vi "test frame felica psk.vi"() -> ()   [LabVIEW 2019]
uses:
  <vilib>/Analysis/3filter.llb/Filter Passband Type.ctl
  <vilib>/addons/Modulation/Analog/controls/Complex Data Waveform.ctl
  <vilib>/addons/Modulation/Analog/support/mod_Set Error Source.vi
  <vilib>/addons/Modulation/Digital/Support/Common/Validators/mod_Generate Filter Coefficients Validate.vi
  <vilib>/addons/Modulation/Digital/General/subVIs/mod_Generate Filter Coefficients.vi
  <vilib>/addons/Modulation/Digital/General/MT Generate PSK System Parameters(M).vi
  <vilib>/Waveform/DWDTOps.llb/DWDT Binary U8 to Digital.vi
  <vilib>/addons/Modulation/Analog/MT Upconvert Baseband (Real).vi
  <vilib>/addons/Modulation/Analog/MT Downconvert Passband (Real).vi
  <vilib>/express/express analysis/Spectral/Block/exnSpectralBlock spectral measurements RMS poly.vi
  <vilib>/express/express analysis/Spectral/Block/exnSpectralBlock spectral measurements RMS WFM.vi
  <vilib>/Analysis/3filter.llb/Butterworth Filter (DBL).vi
  <vilib>/express/express analysis/Spectral/XNode/ExpressSpectralMeasurementsBlockNode.xnode
  <vilib>/addons/Modulation/niDMT.lvlib
  <vilib>/addons/Modulation/niAMT.lvlib
  <vilib>/Analysis/NI_AALBase.lvlib
panel:
  out "Analog signal 4":waveform(dbl)(graph)
  out "spectrum analog signal 5":cluster{"t0":dbl, "dt":dbl, "Y":dbl[]}(graph)
  out "spectrum analog signal 4":cluster{"t0":dbl, "dt":dbl, "Y":dbl[]}(graph)
  out "ripple":dbl format="%.2p"
  out "output array":i16[](array[numeric])
  out "output bit stream":i8[](array[numeric])
  out "Analog signal 3":waveform(dbl)(graph)
  in  "command":enum16{"WUP_REQ"}(ring)
  out "error":i32
  out "spectrum analog signal 3":cluster{"t0":dbl, "dt":dbl, "Y":dbl[]}(graph)
  out "Analog signal 2":waveform(dbl)(graph)
  out "spectrum analog signal 2":cluster{"t0":dbl, "dt":dbl, "Y":dbl[]}(graph)
  out "spectrum analog signal":cluster{"t0":dbl, "dt":dbl, "Y":dbl[]}(graph)
  in  "CARRIER (hz)":dbl
  in  "BIT RATE":dbl
  out "LENGHT":u8[](array[numeric]) format="%x"
  out "dt":dbl
  out "Analog signal":waveform(dbl)(graph)
  out "video signal":cluster{"t0":dbl, "dt":dbl, "Y":dbl[]}(graph)
  out "Digital SIGNAL":digitalwaveform(graph)
  out "CRC":u8[](array[numeric]) format="%x"
  in  "Data":u8[](array[numeric]) format="%x"
  in  "SYNC":u8[](array[numeric]) format="%x"
  in  "Preambula":u8[](array[numeric]) format="%x"
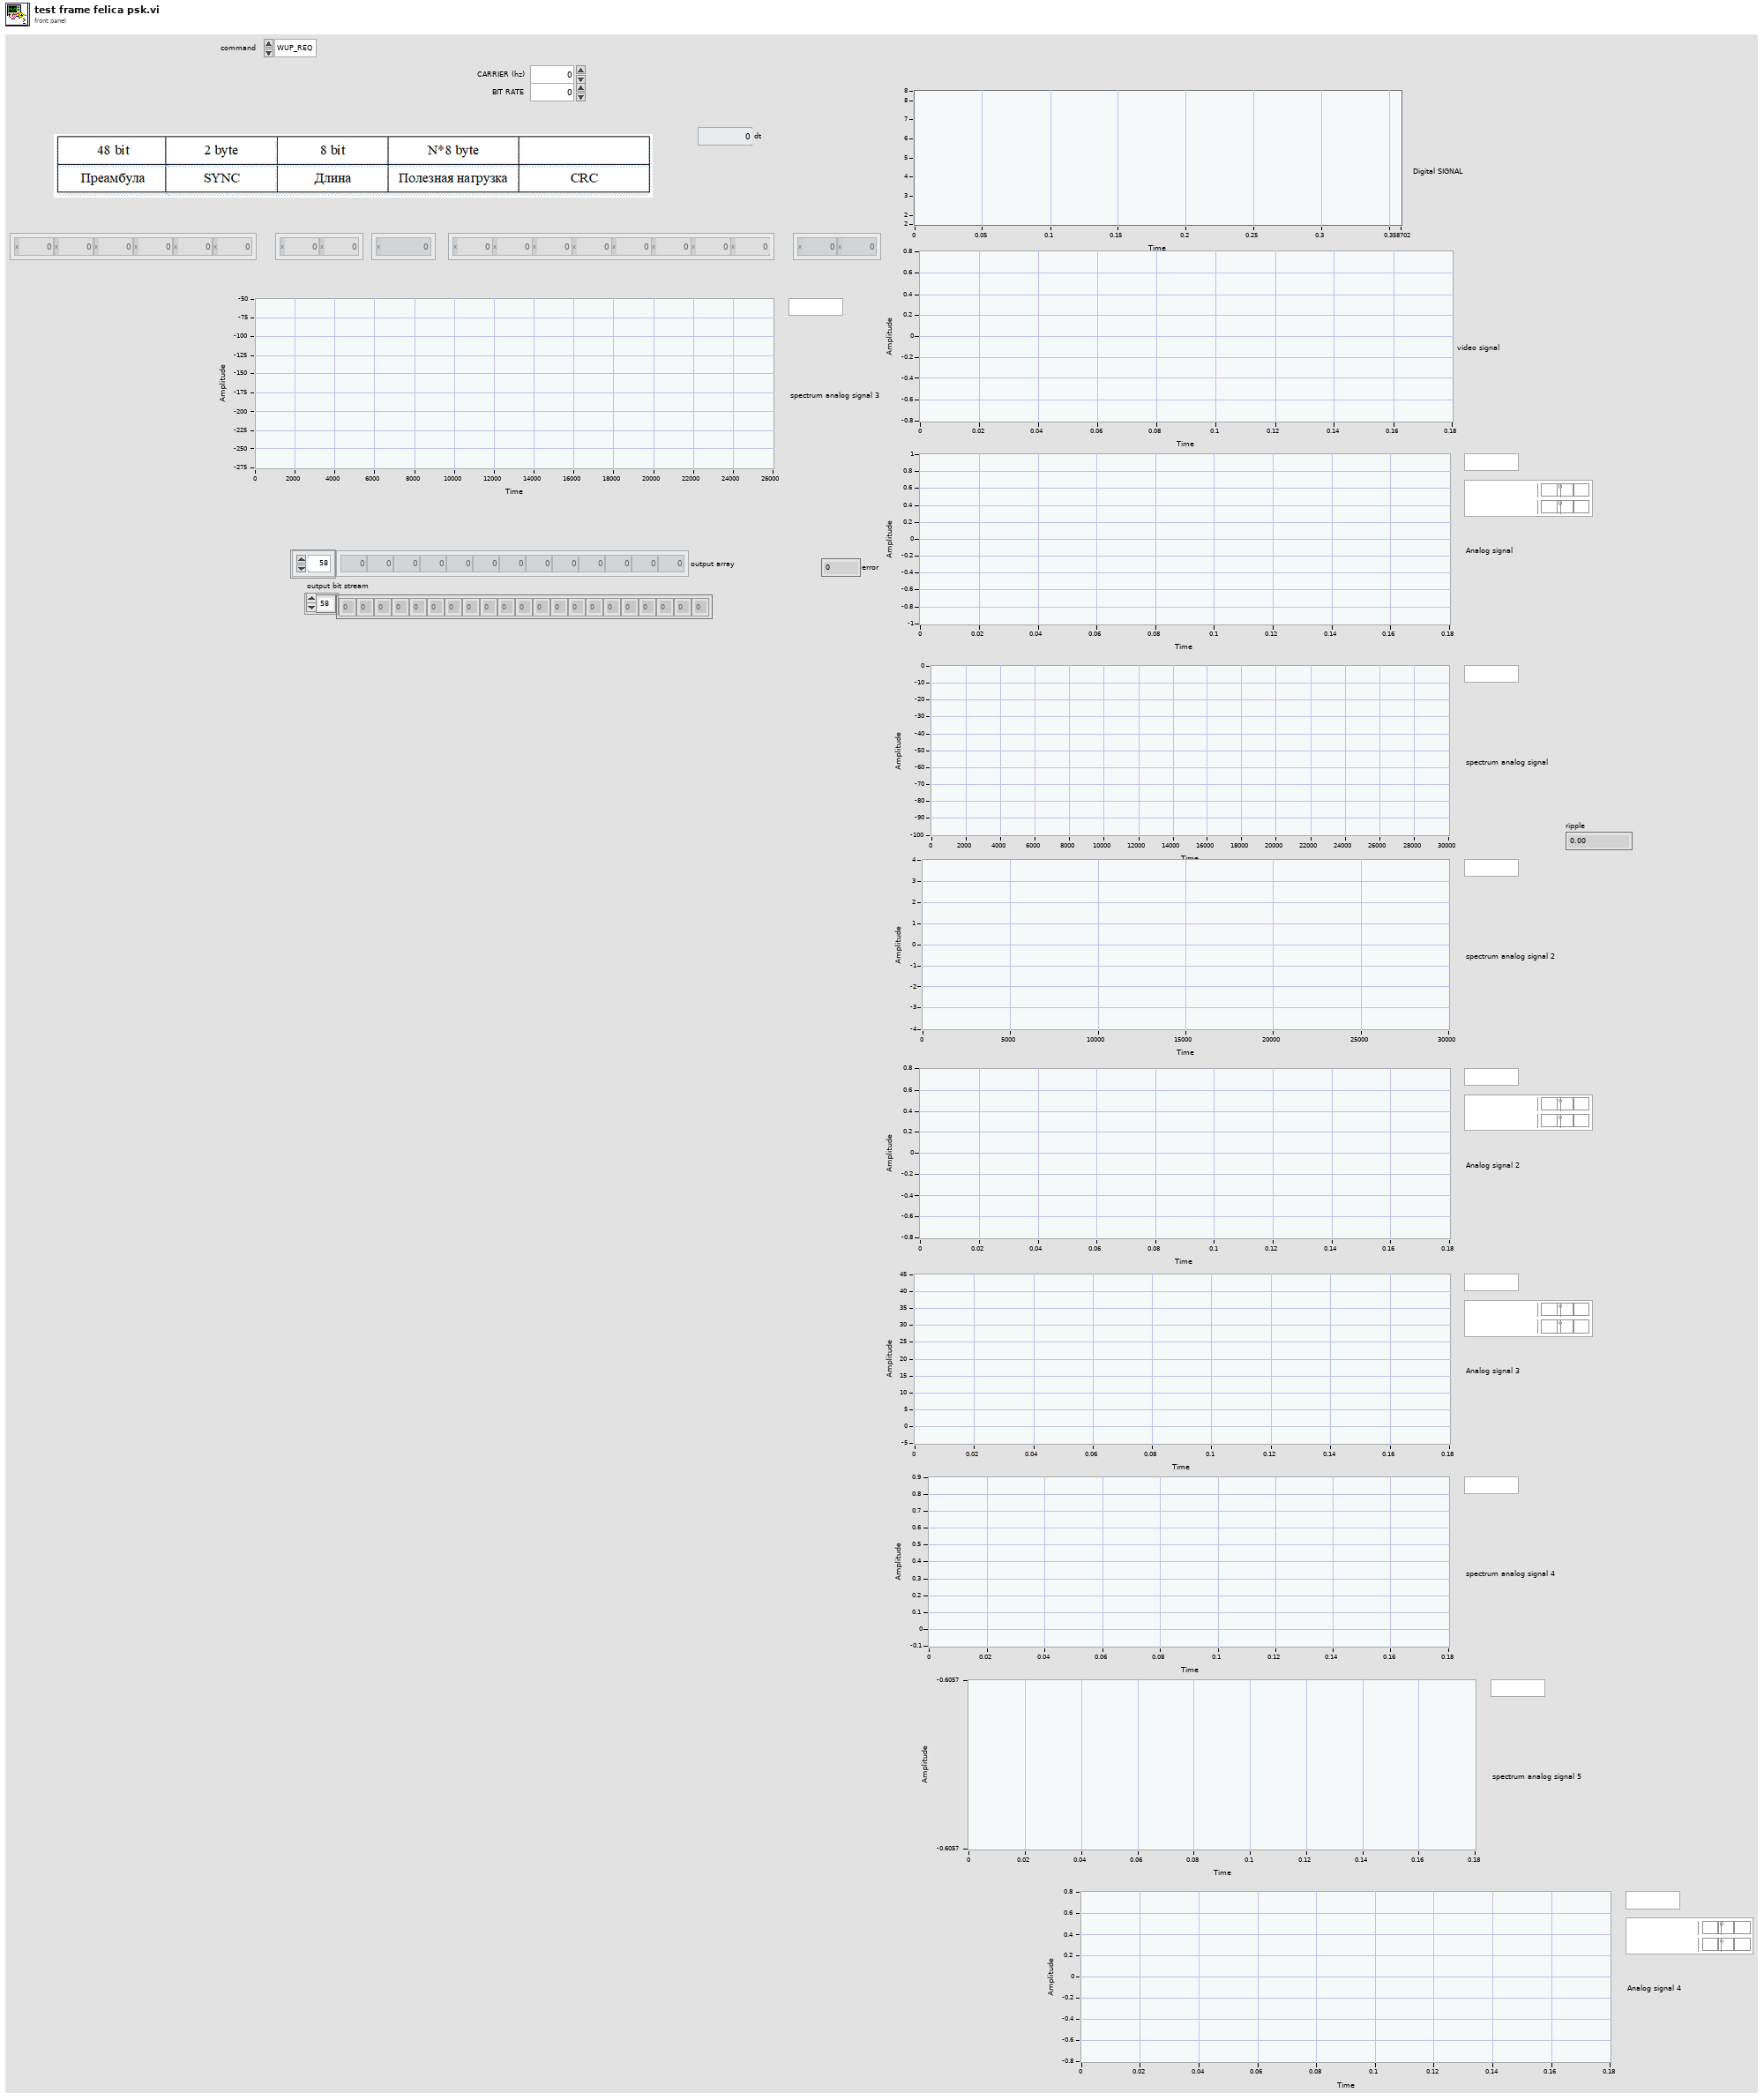
[diagram p1: front panel]
types:
  T1 = cluster{"passband ripple (dB)":dbl, "stopband start (Hz)":dbl, "stopband gain (dB)":dbl, "compute filter stopband ? (T)":bool}
  T2 = enum16{"none", "Raised Cosine", "Root Raised Cos", "Gaussian"}
  T3 = enum16{"FSK", "PSK", "QAM", "MSK", "PAM", "ASK", "CPM"}
  T4 = typedef "niAMT.lvlib/Complex Data Waveform.ctl" = cluster{"t0":dbl, "dt":dbl, "Y":cdb[]}
  T5 = typedef "NI_AALBase.lvlib/Filter Passband Type.ctl" = enum32{"Lowpass", "Highpass", "Bandpass", "Bandstop"}
  T6 = cluster{"samples per symbol (16)":i32, "symbol map":cdb[], "differential PSK":enum16{"disable", "enable"}, "PSK type":u16}
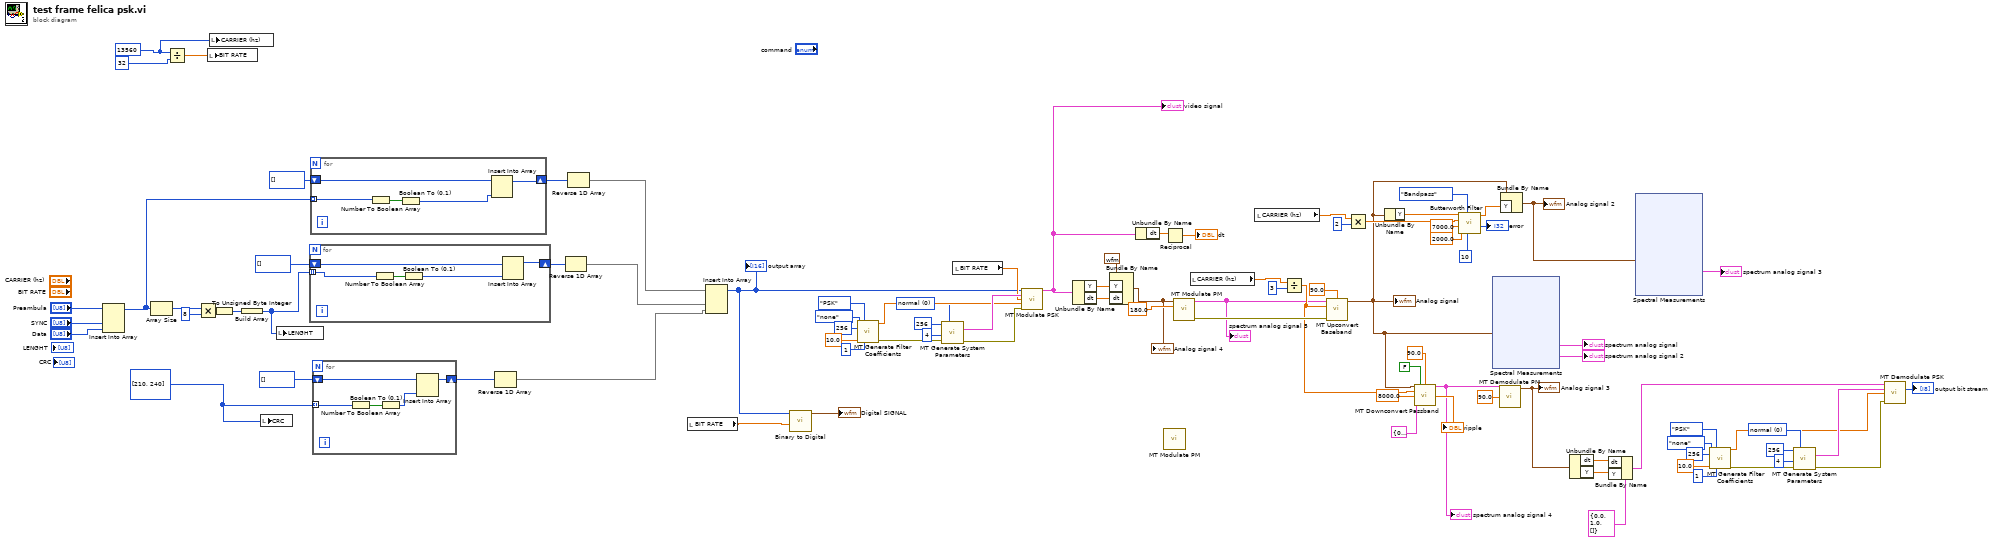
[diagram p0: block diagram]
diagram:
  w10 = u16 0 items=["normal", "shifted", "offset"] ("PSK type")
  w14 = 256 ("pulse shaping samples per symbol (16)")
  w31 = u16 0 items=["normal", "shifted", "offset"] ("PSK type")
  w54 = u32 13560
  w68 = 256 ("pulse shaping samples per symbol (16)")
  w57 = u8[] [210, 240] ("CRC")
  n1 = Insert Into Array(array="Preambula", new element #1="SYNC", new element #2="Data") -> (w86:u8[])  [unwired: 1 in]
  n2 = Array Size(array=w86) -> (size(s)=w85:i32)
  n3 = Divide(x=w54, y=u32 32) -> (x/y=w59:dbl)
  n4 = Multiply(x=w85, y=8) -> (x*y=w83:i32)
  n5 = local write "BIT RATE"(w59) -> ()
  n6 = local write "CARRIER (hz)"(w54) -> ()
  n7 = To Unsigned Byte Integer(number=w83) -> (unsigned 8bit integer=w82:u8)
  n8 = Build Array(w82) -> (w56:u8[])
  n9 = local write "CRC"(w57) -> ()
  n10 = local write "LENGHT"(w56) -> ()
  n11 = for {
    tunnel: w56 -> [w96] mode=indexing
    shift-right: [w94] -> w79
    shift-left: i16[] [] -> [w93]
    n12 = Number To Boolean Array(number=w96) -> (Boolean array=w97:bool[])
    n13 = Boolean To (0,1)(Boolean=w97) -> (0, 1=w95:i16[])
    n14 = Insert Into Array(array=w93, new element=w95) -> (w94:i16[])  [unwired: 1 in]
  }
  n15 = for {
    tunnel: w86 -> [w102] mode=indexing
    shift-right: [w99] -> w87
    shift-left: i16[] [] -> [w98]
    n16 = Number To Boolean Array(number=w102) -> (Boolean array=w101:bool[])
    n17 = Boolean To (0,1)(Boolean=w101) -> (0, 1=w100:i16[])
    n18 = Insert Into Array(array=w98, new element=w100) -> (w99:i16[])  [unwired: 1 in]
  }
  n19 = for {
    tunnel: w57 -> [w104] mode=indexing
    shift-right: [w106] -> w80
    shift-left: i16[] [] -> [w103]
    n20 = Number To Boolean Array(number=w104) -> (Boolean array=w107:bool[])
    n21 = Boolean To (0,1)(Boolean=w107) -> (0, 1=w105:i16[])
    n22 = Insert Into Array(array=w103, new element=w105) -> (w106:i16[])  [unwired: 1 in]
  }
  n23 = Reverse 1D Array(array=w80) -> (reversed array=w76:i16[])
  n24 = Reverse 1D Array(array=w79) -> (reversed array=w78:i16[])
  n25 = Reverse 1D Array(array=w87) -> (reversed array=w77:i16[])
  n26 = local read "BIT RATE"() -> (w58:dbl)
  n27 = Insert Into Array(array=w77, new element #1=w78, new element #2=w76) -> (w30:i16[])  [unwired: 1 in]
  "output array" <- w30
  n28 = call-poly <vilib>:"Binary to Digital.vi"("sample rate"=w58, "binary array"=w30) -> ("digital waveform"=→"Digital SIGNAL":digitalwaveform)  [unwired: 8 in, 1 out]
  n29 = call <vilib>:"MT Generate Filter Coefficients.vi"("pulse shaping filter (none)"=T2."none", "modulation type"=T3."PSK", "pulse shaping samples per symbol (16)"=w68, "matched samples per symbol (16)"=w68, "filter parameter"=10.0, "filter length (symbols)"=1) -> ("pulse shaping filter coefficients"=w66:dbl[], "error out"=w71:errorcluster)  [unwired: 1 in, 7 out]
  n30 = call-poly <vilib>:"MT Generate System Parameters.vi"("samples per symbol (16)"=256, "PSK type"=w31, "M-PSK (4)"=4, "error in (no error)"=w71) -> ("PSK system parameters"=w74:T6, "error out"=w73:errorcluster)  [unwired: 1 in, 9 out]
  n31 = local read "BIT RATE"() -> (w55:dbl)
  n32 = call <vilib>:"MT Modulate PSK.vi"("input bit stream"=w30, "PSK system parameters"=w74, "symbol rate (Hz)"=w55, "pulse shaping filter coefficients"=w66, "error in (no error)"=w73) -> ("output complex waveform"=w51:T4)  [unwired: 8 in, 2 out]
  "video signal" <- w51
  n33 = Unbundle By Name(w51) -> ("Y"=w50:cdb[], "dt"=w48:dbl)
  n34 = Bundle By Name(cluster=waveform(cdb) {"t0"=timestamp(0 s since 1904-01-01), "dt"=1.0, "Y"=[]} ("waveform"), "Y"=w50, "dt"=w48) -> (w1:waveform(cdb))
  "Analog signal 4" <- w1
  n35 = Unbundle By Name(w51) -> ("dt"=w63:dbl)
  n36 = call <vilib>:"MT Modulate PM.vi"() -> ()  [unwired: 14 in, 2 out]
  n37 = Reciprocal(x=w63) -> (1/x=→"dt":dbl)
  n38 = call <vilib>:"MT Modulate PM.vi"("message signal"=w1, "phase deviation (deg)"=180.0 ("modulation index")) -> ("PM modulated waveform"=w2:cluster{"t0":dbl, "dt":dbl, "Y":cdb[]}, "error out"=w52:errorcluster)  [unwired: 12 in]
  "spectrum analog signal 5" <- w2
  n39 = local read "CARRIER (hz)"() -> (w53:dbl)
  n40 = local read "CARRIER (hz)"() -> (w43:dbl)
  n41 = Divide(x=w53, y=u32 3) -> (x/y=w28:dbl)
  n42 = call-poly <vilib>:"MT Upconvert Baseband.vi"("baseband waveform (complex)"=w2, "initial phase (deg)"=90.0, "carrier frequency (Hz)"=w28, "error in (no error)"=w52) -> ("passband waveform"=w29:waveform(dbl))  [unwired: 10 in, 1 out]
  "Analog signal" <- w29
  n43 = Multiply(x=w43, y=u32 2) -> (x*y=w41:dbl)
  n44 = Unbundle By Name(w29) -> ("Y"=w44:dbl[])
  n45 = call-poly <vilib>:"MT Downconvert Passband.vi"("Waveform"=w29, "reset? (F)"=FALSE, "initial phase (deg)"=90.0, "carrier frequency (Hz)"=w28, "passband bandwidth (Hz)"=8000.0, "advanced filter parameters"=T1 {"passband ripple (dB)"=0.01, "stopband start (Hz)"=0.0, "stopband gain (dB)"=-96.0, "compute filter stopband ? (T)"=TRUE}) -> ("downconverted waveform (complex baseband)"=w3:T4, "ripple"=→"ripple":dbl)  [unwired: 6 in, 2 out]
  "spectrum analog signal 4" <- w3
  n46 = call-poly <vilib>:"Butterworth Filter.vi"("order"=10, "filter type"=Filter_Passband_Type."Bandpass", "low cutoff freq: fl"=2000.0, "high cutoff freq: fh"=7000.0, "sampling freq: fs"=w41, "X"=w44) -> ("error"=→"error":i32, "Filtered X"=w40:dbl[])  [unwired: 2 in]
  n47 = xnode "Spectral Measurements"("Signals"=w29) -> ("FFT - (RMS)"=→"spectrum analog signal":cluster{"f0":dbl, "df":dbl, "magnitude":dbl[]}, "Phase"=→"spectrum analog signal 2":cluster{"f0":dbl, "df":dbl, "phase":dbl[]})  [unwired: 1 in, 1 out]
  n48 = call <vilib>:"MT Demodulate PM.vi"("PM modulated waveform"=w3, "phase deviation (deg)"=90.0) -> ("PM demodulated waveform"=w21:waveform(dbl))  [unwired: 11 in, 2 out]
  "Analog signal 3" <- w21
  n49 = Bundle By Name(cluster=w29, "Y"=w40) -> (w37:waveform(dbl))
  "Analog signal 2" <- w37
  n50 = Unbundle By Name(w21) -> ("dt"=w19:dbl, "Y"=w20:dbl[])
  n51 = Bundle By Name(cluster=T4 {"t0"=0.0, "dt"=1.0, "Y"=[]} ("input cluster"), "dt"=w19, "Y"=w20) -> (w22:T4)
  n52 = xnode "Spectral Measurements"("Signals"=w37) -> ("FFT - (RMS)"=→"spectrum analog signal 3":cluster{"f0":dbl, "df":dbl, "magnitude":dbl[]})  [unwired: 1 in, 2 out]
  n53 = call <vilib>:"MT Generate Filter Coefficients.vi"("pulse shaping filter (none)"=T2."none", "modulation type"=T3."PSK", "pulse shaping samples per symbol (16)"=w14, "matched samples per symbol (16)"=w14, "filter parameter"=10.0, "filter length (symbols)"=1) -> ("pulse shaping filter coefficients"=w8:dbl[], "error out"=w17:errorcluster)  [unwired: 1 in, 7 out]
  n54 = call-poly <vilib>:"MT Generate System Parameters.vi"("samples per symbol (16)"=256, "PSK type"=w10, "M-PSK (4)"=4, "error in (no error)"=w17) -> ("PSK system parameters"=w9:T6, "error out"=w7:errorcluster)  [unwired: 1 in, 9 out]
  n55 = call <vilib>:"MT Demodulate PSK.vi"("input complex waveform"=w22, "PSK system parameters"=w9, "matched filter coefficients"=w8, "error in (no error)"=w7) -> ("output bit stream"=→"output bit stream":i8[])  [unwired: 7 in, 4 out]
